vi "NotifyObserver.vi"(8 "error in (no error)":errorcluster, 10 "Variant":variant, 11 "Food in":refnum<class "Food.lvclass">) -> (0 "error out":errorcluster, 3 "Food out":refnum<class "Food.lvclass">)   [LabVIEW 2013, in "Food.lvclass"]
uses:
  Food.lvclass
  Observable.lvclass/Observable.lvclass
  Food.lvclass/Food.ctl
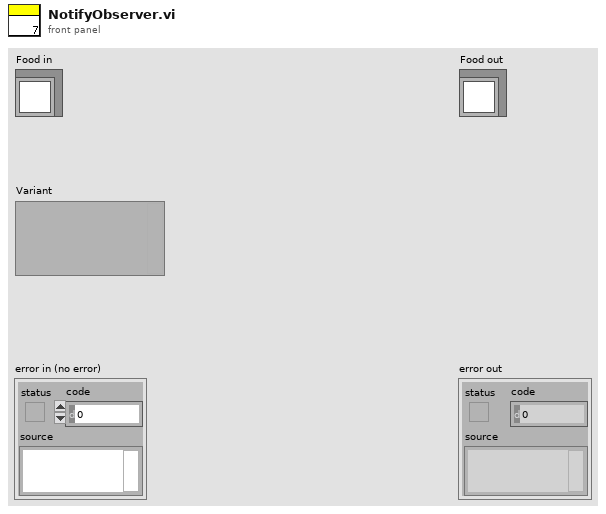
[diagram p1: front panel]
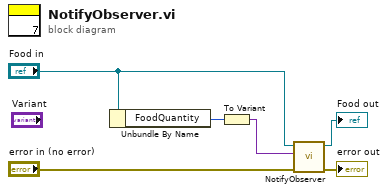
[diagram p0: block diagram]
diagram:
  n1 = Unbundle By Name("Food in") -> ("FoodQuantity"=w2:i32)
  n2 = To Variant(anything=w2) -> (Variant=w1:variant)
  n3 = call-parent "NotifyObserver.vi"("error in (no error)"="error in (no error)", "Variant"=w1, "Observable in"="Food in") -> ("error out"=→"error out":errorcluster, "Observable out"=→"Food out":refnum<class "Food.lvclass">)  [unwired: 7 in]
